vi "ExSimpleFocus.vi"() -> ()   [LabVIEW 2010]
panel:
  in  "stop":bool
  out "Intensity Graph":u16[][](graph)
  in  "Exposure":dbl=0.001 format="%.3f"
  in  "Close Compensation time ms 2":u32=8
  in  "Open Compensation time ms":u32=8
  in  "Temperature":dbl format="%.2f"
  out "error out":errorcluster
  in  "error in (no error)":errorcluster
  # "Note: for the Cascade and\nPhotonMax the open/close\n compensation should be 0"
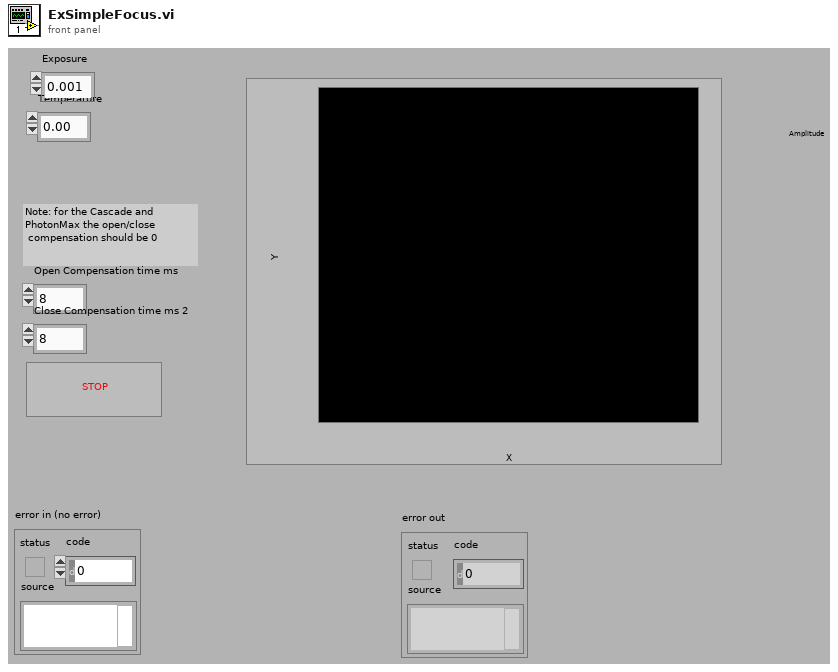
[diagram p1: front panel]
types:
  T1 = cluster{"Open Compensation time ms":u32, "Close Compensation time ms 2":u32}
  T2 = cluster{"Camera Handle":u32, "File Handle":u32, "Image Handle":u32}
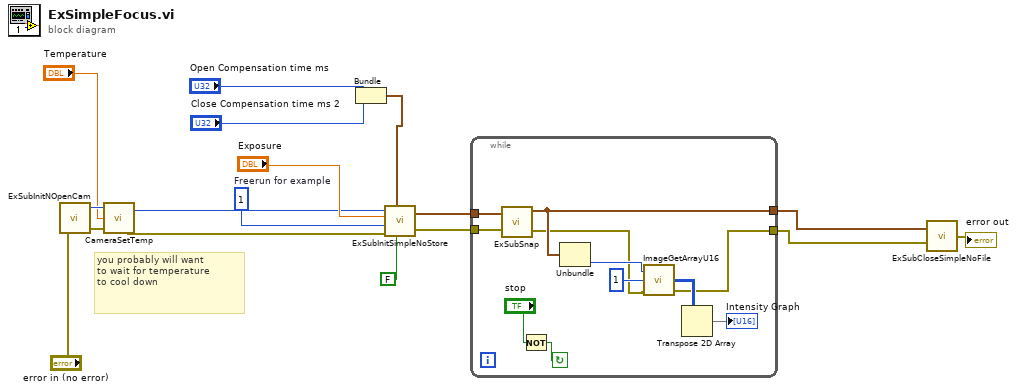
[diagram p0: block diagram]
diagram:
  w4 = 1  # Freerun for example
  # "you probably will want \nto wait for temperature \nto cool down"
  n1 = call "ExSubInitNOpenCam.vi"("error in (no error)"="error in (no error)") -> ("Camera Handle"=w15:u32, "error out"=w16:errorcluster)
  n2 = call <userlib>:"CameraSetTemp.vi"("error in (no error)"=w16, "Temperature"="Temperature", "Camera Handle"=w15) -> ("error out"=w10:errorcluster, "Camera Handle"=w3:u32)
  n3 = Bundle("Open Compensation time ms"="Open Compensation time ms", "Close Compensation time ms 2"="Close Compensation time ms 2") -> (w7:T1)  [unwired: 1 in]
  n4 = call "ExSubInitSimpleNoStore.vi"("Intensifier"=FALSE, "Shutter Comp"=w7, "error in (no error)"=w10, "Triggering mode"=w4, "Exposure"="Exposure", "Camera Handle"=w3) -> ("error out"=w11:errorcluster, "Handles"=w12:cluster{"Camera":u32, "File":u32, "Image":u32})
  n5 = while {
    tunnel: w12 -> [w28]
    tunnel: w11 -> [w27]
    tunnel: [w21] -> w2
    tunnel: [w18] -> w1
    stop <- w26 continue-if-true
    n6 = call "ExSubSnap.vi"("error in (no error)"=w27, "Handle Cluster"=w28) -> ("error out"=w19:errorcluster, "Handle Cluster Out"=w21:T2)
    n7 = Not(x="stop") -> (.not. x?=w26:bool)
    n8 = Unbundle(w21) -> ("Image Handle"=w20:u32)  [unwired: 2 out]
    n9 = call <userlib>:"ImageGetArrayU16.vi"("error in"=w19, "Z position"=1, "Image Handle"=w20) -> ("error out"=w18:errorcluster, "Array uint 16"=w23:u16[][])  [unwired: 1 out]
    n10 = Transpose 2D Array(2D array=w23) -> (transposed array=→"Intensity Graph":u16[][])
  }
  n11 = call "ExSubCloseSimpleNoFile.vi"("error in (no error)"=w1, "Handles In"=w2) -> ("error out"=→"error out":errorcluster)
